vi "buzzer check.vi"() -> ()   [LabVIEW 2017]
panel:
  in  "stop":bool
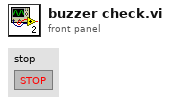
[diagram p1: front panel]
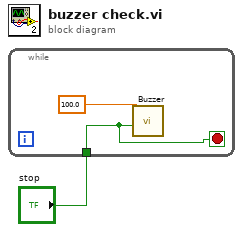
[diagram p0: block diagram]
diagram:
  n1 = while {
    tunnel: "stop" -> [w2]
    stop <- w2 stop-if-true
    n2 = call "Buzzer.vi"("stop"=w2, "frequency [Hz]"=100.0) -> ()  [unwired: 10 in]
  }
